vi "Unit Test.vi"() -> ()   [LabVIEW 2016, in "Instrument.OxfordVRM.lvclass"]
uses:
  Instrument.OxfordVRM.lvclass
  <userlib>/LevyLab/Levylab Instruments/Instrument Types/Cryostat/Typedefs/Magnet Axis--Enum.ctl
  <vilib>/addons/_JKI Toolkits/Caraya/classes/Test/Test.lvclass
  <userlib>/LevyLab/Levylab Instruments/Instrument Types/Cryostat/Instrument.Cryostat.lvclass
panel:
  out "Status Z":string
  out "Status Y":string
  out "Status X":string
  out "error out":errorcluster
  out "Instrument.OxfordVRM out":refnum<class "Instrument.OxfordVRM.lvclass">
  in  "Instrument.OxfordVRM in":refnum<class "Instrument.OxfordVRM.lvclass">
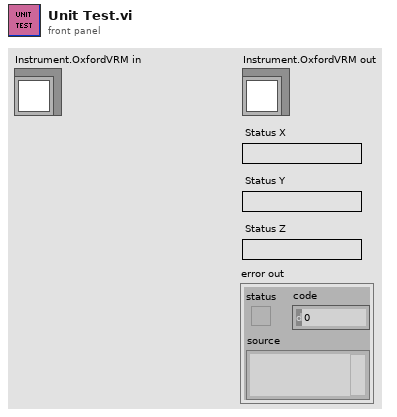
[diagram p1: front panel]
types:
  T1 = typedef "Instrument.Cryostat.lvclass/Magnet Axis--Enum.ctl" = enum16{"Z", "X", "Y"}
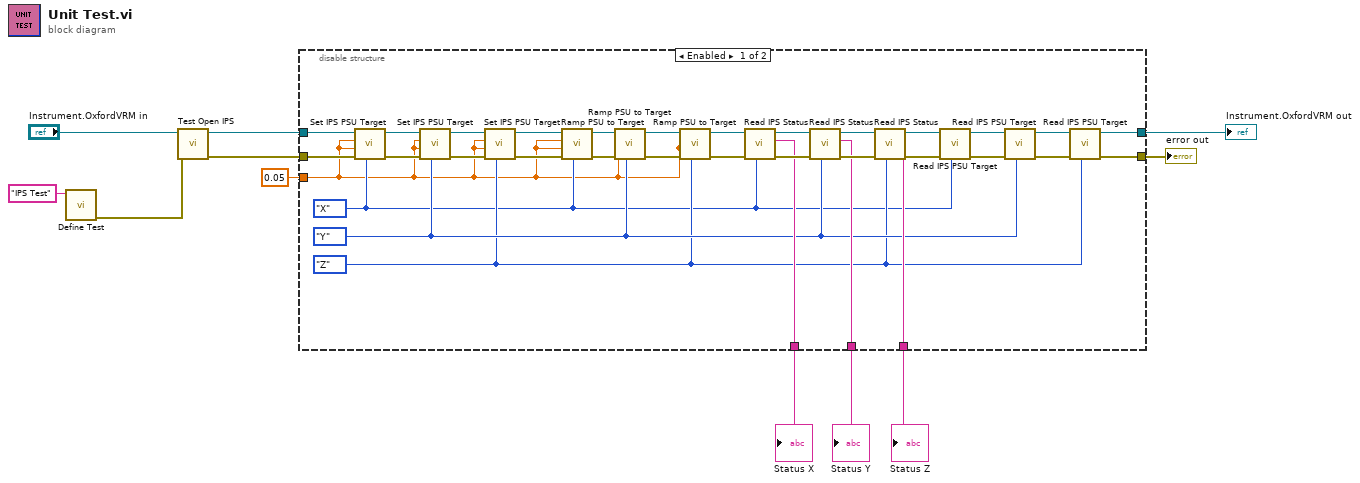
[diagram p0: block diagram]
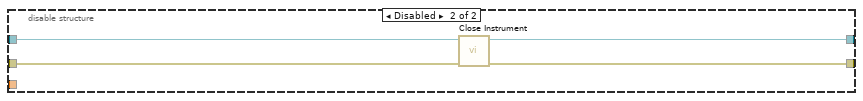
[diagram p2: hidden frame]
diagram:
  n1 = call <vilib>:"Define Test.vi"("Label (VI Title)"="IPS Test") -> ("error out"=w1:errorcluster)  [unwired: 10 in]
  n2 = call "Test Open IPS.vi"("error in (no error)"=w1, "Instrument.OxfordVRM in"="Instrument.OxfordVRM in") -> ("error out"=w4:errorcluster, "Instrument.OxfordVRM out"=w10:refnum<class "Instrument.OxfordVRM.lvclass">)  [unwired: 8 in]
  n3 = disable-structure "Diagram Disable Structure" shown="Enabled" {
    disable-tunnel: w10 -> [w44 w48]
    disable-tunnel: [w31 _] -> w9
    disable-tunnel: [w30 _] -> w8
    disable-tunnel: [w29 _] -> w7
    disable-tunnel: [w20 w46] -> w6
    disable-tunnel: [w21 w47] -> w5
    disable-tunnel: w4 -> [w26 w45]
    disable-tunnel: 0.05 ("Target Field (T)") -> [w12 _]
    frame Enabled {
      w18 = Magnet_Axis--Enum."Z" ("Axis")
      w19 = Magnet_Axis--Enum."Y" ("Axis")
      w13 = Magnet_Axis--Enum."X" ("Axis")
      n4 = call "Set IPS PSU Target.vi"("Axis"=w13, "error in (no error)"=w26, "Target Field Rate (T/min)"=w12, "Target Field (T)"=w12, "Instrument.OxfordVRM in"=w44) -> ("error out"=w38:errorcluster, "Instrument.OxfordVRM out"=w39:refnum<class "Instrument.OxfordVRM.lvclass">)  [unwired: 4 in, 1 out]
      n5 = call "Set IPS PSU Target.vi"("Axis"=w19, "error in (no error)"=w38, "Target Field Rate (T/min)"=w12, "Target Field (T)"=w12, "Instrument.OxfordVRM in"=w39) -> ("error out"=w37:errorcluster, "Instrument.OxfordVRM out"=w40:refnum<class "Instrument.OxfordVRM.lvclass">)  [unwired: 4 in, 1 out]
      n6 = call "Set IPS PSU Target.vi"("Axis"=w18, "error in (no error)"=w37, "Target Field Rate (T/min)"=w12, "Target Field (T)"=w12, "Instrument.OxfordVRM in"=w40) -> ("error out"=w17:errorcluster, "Instrument.OxfordVRM out"=w16:refnum<class "Instrument.OxfordVRM.lvclass">)  [unwired: 4 in, 1 out]
      n7 = call "Ramp PSU to Target.vi"("Axis"=w13, "error in (no error)"=w17, "Target Rate (T/min)"=w12, "Target Field (T)"=w12, "Instrument.OxfordVRM in"=w16) -> ("error out"=w14:errorcluster, "Instrument.OxfordVRM out"=w15:refnum<class "Instrument.OxfordVRM.lvclass">)  [unwired: 5 in]
      n8 = call "Ramp PSU to Target.vi"("Axis"=w19, "error in (no error)"=w14, "Target Rate (T/min)"=w12, "Target Field (T)"=w12, "Instrument.OxfordVRM in"=w15) -> ("error out"=w36:errorcluster, "Instrument.OxfordVRM out"=w41:refnum<class "Instrument.OxfordVRM.lvclass">)  [unwired: 5 in]
      n9 = call "Ramp PSU to Target.vi"("Axis"=w18, "error in (no error)"=w36, "Target Rate (T/min)"=w12, "Target Field (T)"=w12, "Instrument.OxfordVRM in"=w41) -> ("error out"=w35:errorcluster, "Instrument.OxfordVRM out"=w42:refnum<class "Instrument.OxfordVRM.lvclass">)  [unwired: 5 in]
      n10 = call "Read IPS Status.vi"("Axis"=w13, "error in (no error)"=w35, "Instrument.OxfordVRM in"=w42) -> ("error out"=w34:errorcluster, "Status"=w31:string, "Instrument.OxfordVRM out"=w43:refnum<class "Instrument.OxfordVRM.lvclass">)  [unwired: 6 in]
      n11 = call "Read IPS Status.vi"("Axis"=w19, "error in (no error)"=w34, "Instrument.OxfordVRM in"=w43) -> ("error out"=w32:errorcluster, "Status"=w30:string, "Instrument.OxfordVRM out"=w33:refnum<class "Instrument.OxfordVRM.lvclass">)  [unwired: 6 in]
      n12 = call "Read IPS Status.vi"("Axis"=w18, "error in (no error)"=w32, "Instrument.OxfordVRM in"=w33) -> ("error out"=w27:errorcluster, "Status"=w29:string, "Instrument.OxfordVRM out"=w28:refnum<class "Instrument.OxfordVRM.lvclass">)  [unwired: 6 in]
      n13 = call "Read IPS PSU Target.vi"("Axis"=w13, "error in (no error)"=w27, "Instrument.OxfordVRM in"=w28) -> ("error out"=w24:errorcluster, "Instrument.OxfordVRM out"=w25:refnum<class "Instrument.OxfordVRM.lvclass">)  [unwired: 5 in, 2 out]
      n14 = call "Read IPS PSU Target.vi"("Axis"=w19, "error in (no error)"=w24, "Instrument.OxfordVRM in"=w25) -> ("error out"=w22:errorcluster, "Instrument.OxfordVRM out"=w23:refnum<class "Instrument.OxfordVRM.lvclass">)  [unwired: 5 in, 2 out]
      n15 = call "Read IPS PSU Target.vi"("Axis"=w18, "error in (no error)"=w22, "Instrument.OxfordVRM in"=w23) -> ("error out"=w20:errorcluster, "Instrument.OxfordVRM out"=w21:refnum<class "Instrument.OxfordVRM.lvclass">)  [unwired: 5 in, 2 out]
    }
    frame Disabled {
      n16 = call-dynamic "Close Instrument.vi"("error in (no error)"=w45, "Instrument.OxfordVRM in"=w48) -> ("error out"=w46:errorcluster, "Instrument.OxfordVRM out"=w47:refnum<class "Instrument.OxfordVRM.lvclass">)  [unwired: 8 in]
    }
  }
  "Instrument.OxfordVRM out" <- w5
  "error out" <- w6
  "Status X" <- w9
  "Status Y" <- w8
  "Status Z" <- w7
